vi "Evaluate.vi"(0 "object in":refnum<class "ReceptionAngle.lvclass">, 2 "Point":dbl[](array[numeric]), 3 "Ally?":bool, 4 "GameRef":refnum<data-value>, 5 "error in (no error)":errorcluster) -> (14 "object out":refnum<class "ReceptionAngle.lvclass">, 16 "Evaluation":dbl, 19 "error out":errorcluster)   [LabVIEW 2023, in "ReceptionAngle.lvclass"]
uses:
  ReceptionAngle.lvclass
  Game_class/Game.lvclass
  Game_class/Game.lvclass/Game.ctl
  Game_class/Read Utilities.lvclass.vi
  Utilities_class/Utilities.lvclass
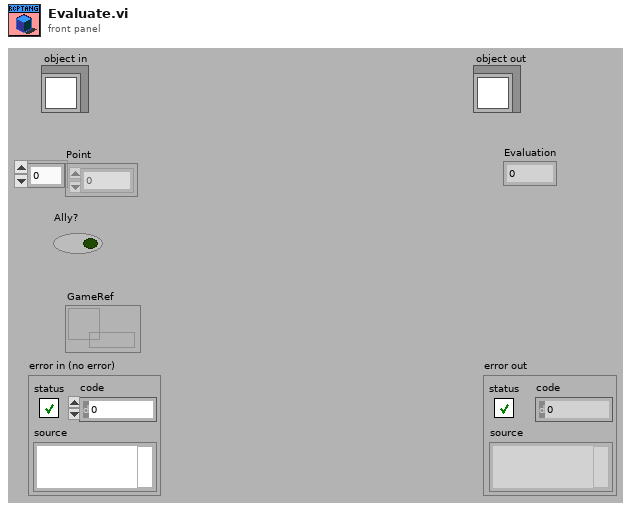
[diagram p1: front panel]
types:
  T1 = typedef "STPParameters.ctl" = cluster{"Skills":T2, "TestSkill":T4, "Events":cluster{"distanceToBallPossession":dbl, "timeForPossessionThreshold":dbl}, "Criteria":cluster{"OpenAngleToGoal":cluster{"minAngle":dbl, "maxAngle":dbl, "minEvaluation":dbl}, "PassDistance":cluster{"maxDistance":dbl, "minDistance":dbl}, "ShotInterception":cluster{"shotSpeed":dbl, "minEnemySpeed":dbl, "minEvaluation":dbl, "maxEnemySpeed":dbl}, "OneTouchShot":cluster{"MaxAngle":dbl, "minEvaluation":dbl}, "PassInterception":cluster{"minEnemySpeed":dbl, "maxEnemySpeed":dbl, "chipPassDistance":dbl, "chipPassEval":dbl, "minEvaluation":dbl}}, "minPassSpeed":dbl, "maxPassSpeed":dbl, "AllyTeamIds":T5[], "ReceiverSpeed":dbl, "minEvaluationToShoot":dbl}
  T2 = typedef "Skills.ctl" = cluster{"CirculateBall":T3, "ProtectBall":cluster{"DistanceFromBall":dbl}}
  T3 = typedef "CIrculateSkillParameters.ctl" = cluster{"rotationAngle":dbl, "velocityFactor":dbl, "OrientationFactor":dbl}
  T4 = typedef "TestSkills.ctl" = enum16{"AlignSkill", "PassSkill", "CirculateBall", "OneTouchShotSkill", "KickToSkill_v2", "ShootSkill", "InterceptBall", "Exit", "GoToSkill_v2"}
  T5 = typedef "AllyTeam.ctl" = enum16{"Keeper", "Defender", "Attacker"}
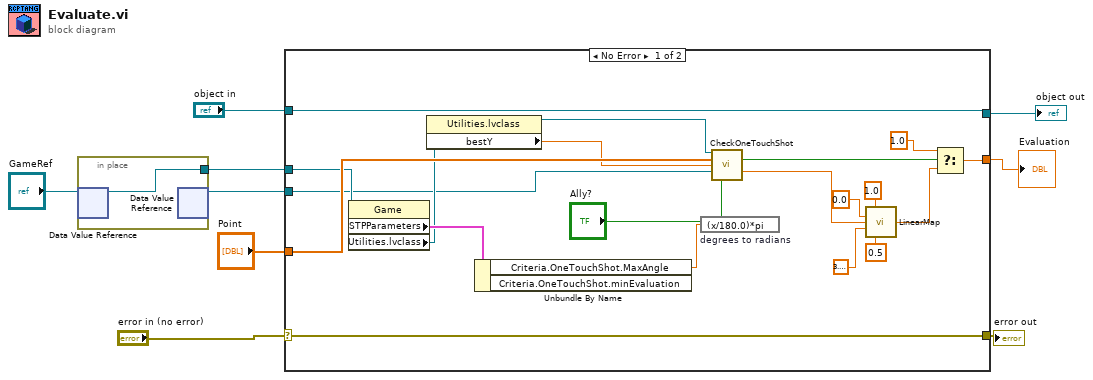
[diagram p0: block diagram]
diagram:
  n1 = in-place {
    in-place-border: [w10] -> w2
    n2 = in-place-dvr #1("GameRef") -> (w10:refnum<class "Game.lvclass">)  [unwired: 1 out]
    n3 = in-place-dvr #1() -> (w1:refnum<data-value>)  [unwired: 1 in, 1 out]
  }
  n4 = case shown="No Error" "error in (no error)" {
    selector: "error in (no error)" -> [w30 w32]
    tunnel: [w30 w32] -> w8
    tunnel: "object in" -> [w23 w31]
    tunnel: [w23 w31] -> w6
    tunnel: w2 -> [w26 _]
    tunnel: "Point" -> [w28 _]
    tunnel: [w13 _] -> w4
    tunnel: w1 -> [w11 _]
    frame No Error {
      n5 = property class="Game"(reference=w26) -> ("STPParameters"=w25:T1, "Utilities.lvclass"=w22:refnum<class "Utilities.lvclass">)  [unwired: 1 in, 2 out]
      n6 = property class="Utilities.lvclass"(reference=w22) -> (reference out=w20:refnum<class "Utilities.lvclass">, "bestY"=w21:dbl)  [unwired: 1 in, 1 out]
      n7 = Unbundle By Name(w25) -> ("Criteria.OneTouchShot.MaxAngle"=w24:dbl)  [unwired: 1 out]
      n8 = expression code="(x/180.0)*pi" "degrees to radians"(w24) -> ()  [unwired: 1 out]
      n9 = call-dynamic "CheckOneTouchShot.vi"("Utilities in"=w20, "Point"=w28, "Best y"=w21, "GameRef"=w11, "Ally?"="Ally?") -> ("OneTouch"=w27:bool, "Angle"=w16:dbl)  [unwired: 7 in, 2 out]
      n10 = call "LinearMap.vi"("MaxY"=1.0, "MaxX"=0.0 ("MaxVal"), "X"=w16, "MinX"=3.141592653589793, "MinY"=0.5) -> ("Y"=w14:dbl)  [unwired: 8 in, 2 out]
      n11 = Select(t=1.0, s=w27, f=w14) -> (s? t:f=w13:dbl)
    }
    frame Error {
    }
  }
  "error out" <- w8
  "object out" <- w6
  "Evaluation" <- w4
